vi "subPortInit.vi"(0 "Control unit ID":i32=1 min=1 max=10) -> (1 "Index":i32, 2 "InitOK":bool)   [LabVIEW 2020]
panel:
  in  "Network port":u16=1200
  in  "ip4":u8 caption="IP address"
  in  "ip3":u8 caption="IP address"
  in  "ip2":u8 caption="IP address"
  in  "ip1":u8 caption="IP address"
  in  "logging on":bool
  in  "Delay":i32(slide) caption="Fast(0)<--->Slow(50)" min=0 max=50 scale=0.0..50.0
  in  "Baudrate":string(combo)="9600"
  in  "Cancel":bool
  in  "OK":bool
  in  "COM port":i32=-1 caption="COMx" min=-1 max=255
  out "Error":i32
  in  "Interface":bool
  # "Parameters of the interface"
  # "COMx=-1: find\nautomatically"
  # "IP=0.0.0.0: connect\n 1. local ip address \n and port 1200"
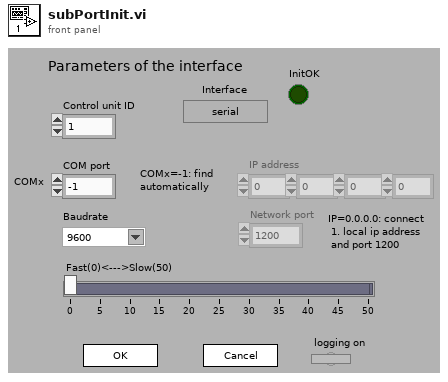
[diagram p1: front panel]
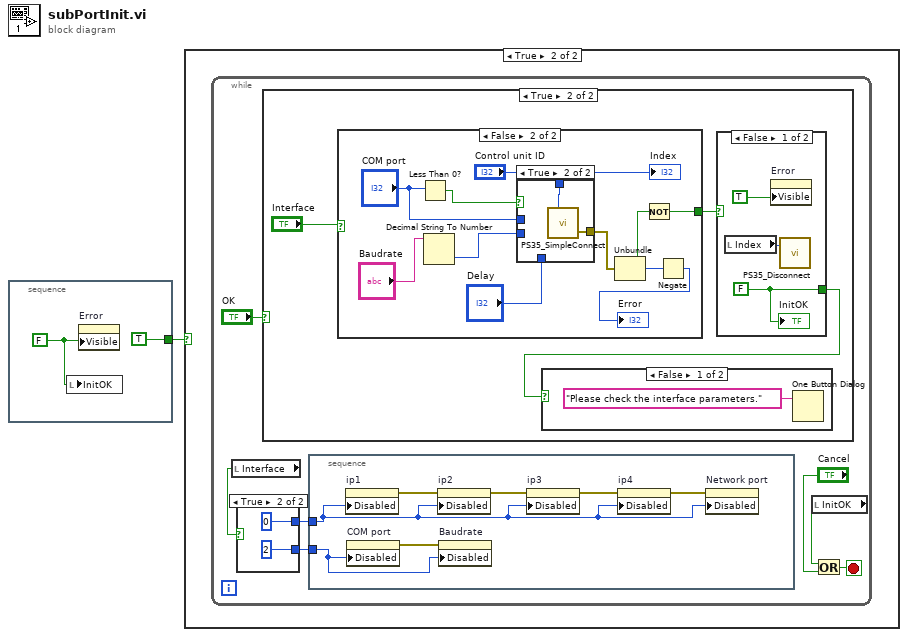
[diagram p0: block diagram]
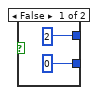
[diagram p3: hidden frame]
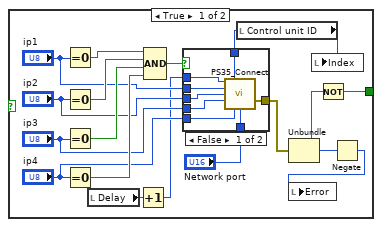
[diagram p5: hidden frame]
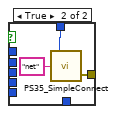
[diagram p6: hidden frame]
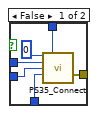
[diagram p7: hidden frame]
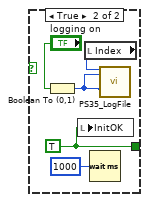
[diagram p8: hidden frame]
diagram:
  n1 = stacked-sequence {
    tunnel: [TRUE] -> w1
    frame #0 {
      w2 = FALSE ("Visible")
      n2 = local write "InitOK"(w2) -> ()
      n3 = property on="Error" class="DigNum (strict)"("Visible"=w2) -> ()  [unwired: 2 in, 2 out]
    }
  }
  n4 = case shown="True" w1 {
    frame False {
    }
    frame True {
      n5 = while {
        stop <- w10 stop-if-true
        n6 = local read "Interface"() -> (w4:bool)
        n7 = case shown="True" w4 {
          tunnel: [0 2] -> w5
          tunnel: [2 0] -> w6
          frame False {
          }
          frame True {
          }
        }
        n8 = case shown="True" "OK" {
          frame False {
          }
          frame True {
            n9 = case shown="False" "Interface" {
              tunnel: [w38 w62] -> w23
              frame True {
                n10 = Equal To 0?(x="ip1") -> (x = 0?=w35:bool)
                n11 = Equal To 0?(x="ip2") -> (x = 0?=w34:bool)
                n12 = Equal To 0?(x="ip3") -> (x = 0?=w32:bool)
                n13 = Equal To 0?(x="ip4") -> (x = 0?=w33:bool)
                n14 = local read "Delay"() -> (w26:i32)
                n15 = Increment(x=w26) -> (x+1=w25:i32)
                n16 = Compound Arithmetic op=AND(w35, w34, w32, w33) -> (w36:bool)
                n17 = local read "Control unit ID"() -> (w42:i32)
                n18 = case shown="False" w36 {
                  tunnel: [w50 w53] -> w39
                  tunnel: w42 -> [w49 w52]
                  tunnel: "ip1" -> [w48 _]
                  tunnel: "ip2" -> [w47 _]
                  tunnel: "ip3" -> [w46 _]
                  tunnel: "ip4" -> [w45 _]
                  tunnel: "Network port" -> [w44 _]
                  tunnel: w25 -> [w43 _]
                  frame False {
                    n19 = call "PS35_Connect.vi"("Interface"=w43, "Control unit ID"=w49, "par1"=w48, "par2"=w47, "par3"=w46, "par4"=w45, "par5"=w44) -> ("error out"=w50:errorcluster)  [unwired: 8 in]
                  }
                  frame True {
                    n20 = call "PS35_SimpleConnect.vi"("Serial number"="net", "Control unit ID"=w52) -> ("error out"=w53:errorcluster)  [unwired: 2 in]
                  }
                }
                n21 = Unbundle(w39) -> ("status"=w40:bool, "code"=w41:i32)  [unwired: 1 out]
                n22 = local write "Index"(w42) -> ()
                n23 = Not(x=w40) -> (.not. x?=w38:bool)
                n24 = Negate(x=w41) -> (-x=w37:i32)
                n25 = local write "Error"(w37) -> ()
              }
              frame False {
                n26 = Less Than 0?(x="COM port") -> (x < 0?=w55:bool)
                n27 = Decimal String To Number(string="Baudrate") -> (number=w58:i32)  [unwired: 2 in, 1 out]
                n28 = case shown="True" w55 {
                  tunnel: [w70 w72] -> w64
                  tunnel: "Control unit ID" -> [w68 w71]
                  tunnel: "COM port" -> [w67 _]
                  tunnel: w58 -> [w66 _]
                  tunnel: "Delay" -> [w65 _]
                  frame False {
                    n29 = call "PS35_Connect.vi"("Interface"=u32 0, "Control unit ID"=w68, "par1"=w67, "par2"=w66, "par3"=w65) -> ("error out"=w70:errorcluster)  [unwired: 10 in]
                  }
                  frame True {
                    n30 = call "PS35_SimpleConnect.vi"("Control unit ID"=w71) -> ("error out"=w72:errorcluster)  [unwired: 3 in]
                  }
                }
                n31 = Unbundle(w64) -> ("status"=w61:bool, "code"=w63:i32)  [unwired: 1 out]
                n32 = Not(x=w61) -> (.not. x?=w62:bool)
                n33 = Negate(x=w63) -> (-x=→"Error":i32)
                "Index" <- "Control unit ID"
              }
            }
            n34 = case shown="False" w23 {
              tunnel: [w73 w77] -> w24
              frame False {
                w73 = FALSE ("WriteOK")
                n35 = local read "Index"() -> (w74:i32)
                n36 = property on="Error" class="DigNum (strict)"("Visible"=TRUE) -> ()  [unwired: 2 in, 2 out]
                n37 = call "PS35_Disconnect.vi"("Control unit ID"=w74) -> ()  [unwired: 2 in, 1 out]
                "InitOK" <- w73
              }
              frame True {
                w77 = TRUE ("WriteOK")
                n38 = Boolean To (0,1)(Boolean="logging on") -> (0, 1=w76:i16)
                n39 = local write "InitOK"(w77) -> ()
                n40 = local read "Index"() -> (w79:i32)
                n41 = Wait (ms)(milliseconds to wait=u32 1000 ("Zu wartende ms")) -> ()  [unwired: 1 out]
                n42 = call "PS35_LogFile.vi"("Control unit ID"=w79, "nOpen"=w76, "Mode"=w76) -> ()  [unwired: 16 in, 1 out]
              }
            }
            n43 = case shown="False" w24 {
              frame False {
                n44 = One Button Dialog(message="Please check the interface parameters.") -> ()  [unwired: 1 in, 1 out]
              }
              frame True {
              }
            }
          }
        }
        n45 = stacked-sequence {
          tunnel: w5 -> [w15]
          tunnel: w6 -> [w17]
          frame #0 {
            n46 = property on="ip1" class="DigNum (strict)"("Disabled"=w17) -> (error out=w18:errorcluster)  [unwired: 2 in, 1 out]
            n47 = property on="COM port" class="DigNum (strict)"("Disabled"=w15) -> (error out=w16:errorcluster)  [unwired: 2 in, 1 out]
            n48 = property on="ip2" class="DigNum (strict)"(error in=w18, "Disabled"=w17) -> (error out=w19:errorcluster)  [unwired: 1 in, 1 out]
            n49 = property on="Baudrate" class="CmbBox"(error in=w16, "Disabled"=w15) -> ()  [unwired: 1 in, 2 out]
            n50 = property on="ip3" class="DigNum (strict)"(error in=w19, "Disabled"=w17) -> (error out=w20:errorcluster)  [unwired: 1 in, 1 out]
            n51 = property on="ip4" class="DigNum (strict)"(error in=w20, "Disabled"=w17) -> (error out=w21:errorcluster)  [unwired: 1 in, 1 out]
            n52 = property on="Network port" class="DigNum (strict)"(error in=w21, "Disabled"=w17) -> ()  [unwired: 1 in, 2 out]
          }
        }
        n53 = local read "InitOK"() -> (w7:bool)
        n54 = Or(x=w7, y="Cancel") -> (x .or. y?=w10:bool)
      }
    }
  }
